vi "HFRR ADV v02.vi"() -> ()   [LabVIEW 2025] (continued)
        n337 = String Length(string=w410) -> (length=w409:i32)
        n338 = Greater?(x=w409, y=1) -> (0:w407:bool)
        n339 = case shown="False" w407 {
          tunnel: w406 -> [w435 _]
          frame False {
            n340 = case shown="False" w435 {
              frame True {
                w436 = "Test Start In Service Mode" ("Tip Strip")
                w437 = T19."Enabled" ("Disabled")
                n341 = property on="Auto Start Test" class="Bool (strict)"("DisabledEnum"=w437, "TipStrip"=w436) -> ()  [unwired: 2 in, 2 out]
                n342 = property on="RUN" class="Bool (strict)"("DisabledEnum"=w437, "TipStrip"=w436) -> ()  [unwired: 2 in, 2 out]
              }
              frame False {
                w438 = "Enter File Name to Start Test" ("Tip Strip")
                w439 = T19."Disabled and Grayed Out" ("Disabled")
                n343 = property on="Auto Start Test" class="Bool (strict)"("DisabledEnum"=w439, "TipStrip"=w438) -> ()  [unwired: 2 in, 2 out]
                n344 = property on="RUN" class="Bool (strict)"("DisabledEnum"=w439, "TipStrip"=w438) -> ()  [unwired: 2 in, 2 out]
              }
            }
          }
          frame True {
            w440 = "" ("Tip Strip")
            w441 = T19."Enabled" ("Disabled")
            n345 = property on="Auto Start Test" class="Bool (strict)"("DisabledEnum"=w441, "TipStrip"=w440) -> ()  [unwired: 2 in, 2 out]
            n346 = property on="RUN" class="Bool (strict)"("DisabledEnum"=w441, "TipStrip"=w440) -> ()  [unwired: 2 in, 2 out]
          }
        }
      }
      event "RUN": Value Change {
        n347 = event-data() -> ()  [unwired: 1 in, 6 out]
        n348 = local read "RUN"() -> (w443:bool)
        n349 = case shown="False" w443 {
          frame False {
            n350 = flat-sequence {
              frame #0 {
                n351 = local write "START TEMP"(FALSE ("START TEMP")) -> ()
              }
              frame #1 {
                n352 = Wait (ms)(milliseconds to wait=u32 1500) -> ()  [unwired: 1 out]
              }
              frame #2 {
                n353 = local write "Humidity 2"(TRUE ("Humidity")) -> ()
              }
              frame #3 {
                n354 = local write "Due Write"("VC;0") -> ()
              }
              frame #4 {
                n355 = Wait (ms)(milliseconds to wait=u32 1500) -> ()  [unwired: 1 out]
              }
              frame #5 {
                w453 = T19."Enabled" ("Disabled")
                (unwired) T25."Imaging" ("Main Dashboard Buttons")
                (unwired) T21."Adv Scar" ("Main Tab")
                w455 = "" ("FILE")
                n356 = local write "measured_stroke"(0.0 ("measured_stroke")) -> ()
                n357 = local write "Due Write"("VC;0") -> ()
                n358 = local write "FILE"(w455) -> ()
                n359 = local write "Batch Ref Num :"(w455) -> ()
                n360 = local write "Fuel Discription :"(w455) -> ()
                n361 = local write "Main Tab"(T4."Adv Scar" ("Main Tab")) -> ()
                n362 = local write "Remarks :"(w455) -> ()
                n363 = local write "Main Dashboard Buttons"(T1."Imaging" ("Main Dashboard Buttons")) -> ()
                n364 = local write "TEST FILE NAM,E SAVED"(FALSE ("TEST FILE NAM,E SAVED")) -> ()
                n365 = property on="Stroke ( mm )" class="WFChart (strict)"("History Data"=cluster{"y":dbl, dbl, "y":dbl}[] []) -> ()  [unwired: 2 in, 2 out]
                n366 = property on="Auto Start Test" class="Bool (strict)"("Visible"=TRUE) -> ()  [unwired: 2 in, 2 out]
                n367 = property on="FRICVALZ 2" class="Bool (strict)"("DisabledEnum"=w453) -> ()  [unwired: 2 in, 2 out]
                n368 = property on="FRICVALZ 4" class="Bool (strict)"("DisabledEnum"=w453) -> ()  [unwired: 2 in, 2 out]
                n369 = property on="FRICVALZ 3" class="Bool (strict)"("DisabledEnum"=w453) -> ()  [unwired: 2 in, 2 out]
              }
            }
          }
          frame True {
            n370 = stacked-sequence {
              frame #0 {
                n371 = local write "FRICVALZ 4"(TRUE ("FRICVALZ 4")) -> ()
                n372 = local write "Due Write"("DAC;200") -> ()
              }
              frame #1 {
              }
              frame #2 {
              }
              frame #3 {
                n373 = Wait (ms)(milliseconds to wait=u32 1000) -> ()  [unwired: 1 out]
              }
              frame #4 {
                n374 = local write "Due Write"("VC;1") -> ()
              }
              frame #5 {
                n375 = Wait (ms)(milliseconds to wait=u32 1000) -> ()  [unwired: 1 out]
              }
              frame #6 {
                n376 = local write "Due Write"("VC;1") -> ()
              }
              frame #7 {
                n377 = Wait (ms)(milliseconds to wait=u32 1500) -> ()  [unwired: 1 out]
              }
              frame #8 {
                w466 = T19."Disabled" ("Disabled")
                n378 = property on="Auto Start Test" class="Bool (strict)"("Visible"=FALSE) -> ()  [unwired: 2 in, 2 out]
                n379 = local write "START TEMP"(TRUE ("START TEMP")) -> ()
                n380 = property on="FRICVALZ 2" class="Bool (strict)"("DisabledEnum"=w466) -> ()  [unwired: 2 in, 2 out]
                n381 = property on="FRICVALZ 4" class="Bool (strict)"("DisabledEnum"=w466) -> ()  [unwired: 2 in, 2 out]
                n382 = property on="FRICVALZ 3" class="Bool (strict)"("DisabledEnum"=w466) -> ()  [unwired: 2 in, 2 out]
              }
            }
          }
        }
      }
      event "run test Calibration": Value Change {
        n383 = event-data() -> ()  [unwired: 1 in, 6 out]
        n384 = local read "run test Calibration"() -> (w468:bool)
        n385 = case shown="False" w468 {
          frame False {
            n386 = flat-sequence {
              frame #0 {
                n387 = local write "START TEMP"(FALSE ("START TEMP")) -> ()
              }
              frame #1 {
                n388 = Wait (ms)(milliseconds to wait=u32 1500) -> ()  [unwired: 1 out]
              }
              frame #2 {
              }
              frame #3 {
                n389 = local write "Due Write"("VC;0") -> ()
              }
              frame #4 {
                n390 = Wait (ms)(milliseconds to wait=u32 1500) -> ()  [unwired: 1 out]
              }
              frame #5 {
                n391 = local write "Due Write"("VC;0") -> ()
                n392 = property on="Tab Control 6" class="TabCtl (strict)"("Visible"=FALSE) -> ()  [unwired: 2 in, 2 out]
                n393 = local write "Friction Force Calibration Result Tab"(enum32{"Calibration Results", "Page 2"}."Calibration Results" ("Friction Force Calibration Result Tab")) -> ()
                n394 = property on="Friction Force Calibration Result Tab" class="TabCtl (strict)"("Visible"=TRUE) -> ()  [unwired: 2 in, 2 out]
              }
            }
          }
          frame True {
            n395 = flat-sequence {
              frame #0 {
                n396 = local write "Due Write"("VC;1") -> ()
              }
              frame #1 {
                n397 = Wait (ms)(milliseconds to wait=u32 1000) -> ()  [unwired: 1 out]
              }
              frame #2 {
                n398 = local write "Due Write"("VC;1") -> ()
              }
              frame #3 {
                n399 = Wait (ms)(milliseconds to wait=u32 2000) -> ()  [unwired: 1 out]
              }
              frame #4 {
                n400 = local write "START TEMP"(TRUE ("START TEMP")) -> ()
                n401 = property on="Tab Control 6" class="TabCtl (strict)"("Visible"=TRUE) -> ()  [unwired: 2 in, 2 out]
                n402 = local write "Friction Force Calibration Result Tab"(enum32{"Calibration Results", "Page 2"}."Calibration Results" ("Friction Force Calibration Result Tab")) -> ()
              }
            }
          }
        }
      }
      event "Auto": Value Change {
        n403 = event-data() -> ()  [unwired: 1 in, 6 out]
        n404 = stacked-sequence {
          frame #0 {
            n405 = local write "FILE"("") -> ()
          }
          frame #1 {
            n406 = Get Date/Time In Seconds() -> (seconds since 1Jan1904=w489:timestamp)
            n407 = Format Into String(format string="%<%m_%d_%Y_%I_%M_%S_%p>T", w489) -> (resulting string=w488:string)  [unwired: 2 in, 1 out]
            n408 = local write "FILE"(w488) -> ()
          }
        }
        n409 = local read "Auto"() -> (w486:bool)
        n410 = Not(x=w486) -> (.not. x?=w485:bool)
        n411 = local write "Auto"(w485) -> ()
      }
      event "Auto Start Temp": Value Change {
        n412 = event-data() -> ()  [unwired: 1 in, 6 out]
        n413 = local read "Auto Start Test"() -> (w492:bool)
        n414 = case shown="False" w492 {
          frame False {
            n415 = stacked-sequence {
              frame #0 {
                n416 = local write "START TEMP"(FALSE ("START TEMP")) -> ()
              }
              frame #1 {
                n417 = Wait (ms)(milliseconds to wait=u32 2000) -> ()  [unwired: 1 out]
              }
              frame #2 {
                n418 = local write "Due Write"("VC;0") -> ()
              }
              frame #3 {
                n419 = Wait (ms)(milliseconds to wait=u32 2000) -> ()  [unwired: 1 out]
              }
              frame #4 {
                w503 = T19."Enabled" ("Disabled")
                (unwired) T25."Imaging" ("Main Dashboard Buttons")
                w504 = "" ("FILE")
                n420 = local write "Main Tab"(T4."Adv Scar" ("Main Tab")) -> ()
                n421 = local write "measured_stroke"(0.0 ("measured_stroke")) -> ()
                n422 = local write "Main Dashboard Buttons"(T1."Imaging" ("Main Dashboard Buttons")) -> ()
                n423 = property on="RUN" class="Bool (strict)"("Visible"=TRUE) -> ()  [unwired: 2 in, 2 out]
                n424 = local write "Due Write"("VC;0") -> ()
                n425 = local write "Humidity 2"(TRUE ("Humidity")) -> ()
                n426 = local write "TEST FILE NAM,E SAVED"(FALSE ("TEST FILE NAM,E SAVED")) -> ()
                n427 = local write "Fuel Discription :"(w504) -> ()
                n428 = local write "Batch Ref Num :"(w504) -> ()
                n429 = local write "Remarks :"(w504) -> ()
                n430 = local write "FILE"(w504) -> ()
                n431 = property on="FRICVALZ 2" class="Bool (strict)"("DisabledEnum"=w503) -> ()  [unwired: 2 in, 2 out]
                n432 = property on="FRICVALZ 4" class="Bool (strict)"("DisabledEnum"=w503) -> ()  [unwired: 2 in, 2 out]
                n433 = property on="FRICVALZ 3" class="Bool (strict)"("DisabledEnum"=w503) -> ()  [unwired: 2 in, 2 out]
              }
            }
          }
          frame True {
            n434 = stacked-sequence {
              frame #0 {
                n435 = local write "Due Write"("DAC;200") -> ()
              }
              frame #1 {
                n436 = Wait (ms)(milliseconds to wait=u32 1000) -> ()  [unwired: 1 out]
              }
              frame #2 {
              }
              frame #3 {
              }
              frame #4 {
                n437 = local write "Due Write"("VC;1") -> ()
              }
              frame #5 {
                n438 = Wait (ms)(milliseconds to wait=u32 1000) -> ()  [unwired: 1 out]
              }
              frame #6 {
                n439 = local write "Due Write"("VC;1") -> ()
              }
              frame #7 {
                n440 = Wait (ms)(milliseconds to wait=u32 1500) -> ()  [unwired: 1 out]
              }
              frame #8 {
                w513 = T19."Disabled" ("Disabled")
                n441 = property on="RUN" class="Bool (strict)"("Visible"=FALSE) -> ()  [unwired: 2 in, 2 out]
                n442 = property on="FRICVALZ 2" class="Bool (strict)"("DisabledEnum"=w513) -> ()  [unwired: 2 in, 2 out]
                n443 = property on="FRICVALZ 4" class="Bool (strict)"("DisabledEnum"=w513) -> ()  [unwired: 2 in, 2 out]
                n444 = property on="FRICVALZ 3" class="Bool (strict)"("DisabledEnum"=w513) -> ()  [unwired: 2 in, 2 out]
                "START TEMP" <- TRUE
              }
            }
          }
        }
      }
      event "FILE", "USERNAME", "USER ID": Mouse Enter {
        n445 = event-data() -> ()  [unwired: 1 in, 4 out]
        n446 = dll-call lib="kernel32.dll" fn="Wow64DisableWow64FsRedirection"("OldValue"=0) -> (error out=w520:errorcluster, "OldValue"=w518:i32)  [unwired: 4 in, 1 out]
        n447 = call <vilib>:"System Exec.vi"("run minimized? (F)"=TRUE, "error in (no error)"=w520, "command line"="C:\\Program Files\\Common Files\\Microsoft Shared\\Ink\\TabTip.exe") -> ("error out"=w519:errorcluster)  [unwired: 5 in, 3 out]
        n448 = dll-call lib="kernel32.dll" fn="Wow64EnableWow64FsRedirection"(error in=w519, "OldValue"=w518) -> ()  [unwired: 4 in, 2 out]
      }
      event "EDIT": Value Change {
        n449 = event-data() -> ()  [unwired: 1 in, 6 out]
        n450 = local read "EDIT"() -> (w521:bool)
        n451 = case shown="False" w521 {
          frame False {
            n452 = control-ref of="This VI"() -> (w538:refnum<vi>)
            n453 = property class="VI"(reference=w538) -> (reference out=w529:refnum<vi>, error out=w533:errorcluster, "Panel"=w537:refnum<vi>)  [unwired: 1 in]
            n454 = property class="Pnl"(reference=w537, error in=w533) -> (reference out=w531:refnum<vi>, error out=w534:errorcluster, "Panes[]"=w536:refnum<vi>[])
            n455 = for {
              tunnel: w536 -> [w544] mode=indexing
              tunnel: T24."Always Off" ("Horizontal Scrollbar Visibility") -> [w543]
              tunnel: w534 -> [w540]
              tunnel: [w539] -> w532
              n456 = property class="Pane"(reference=w544, error in=w540, "HorizScrollbarVisibility"=w543) -> (reference out=w541:refnum<vi>, error out=w542:errorcluster)
              n457 = Close Reference(reference=w541, error in (no error)=w542) -> (error out=w539:errorcluster)
            }
            n458 = Close Reference(reference=w531, error in (no error)=w532) -> (error out=w530:errorcluster)
            n459 = Close Reference(reference=w529, error in (no error)=w530) -> (error out=w524:errorcluster)
            "error out 7" <- w524
            n460 = call <vilib>:"Clear Errors.vi"("error in (no error)"=w524) -> ("error out"=w523:errorcluster)  [unwired: 5 in, 1 out]
            n461 = local write "Service Password enable"(FALSE ("Service Password enable")) -> ()
            n462 = call <userlib>:"Fit VI window to Largest Dec.vi"("error in (no error)"=w523, "border spacing (2 px)"=1) -> ("error out"=w528:errorcluster, "dup VI Ref"=w526:refnum<vi>)  [unwired: 4 in]
            n463 = invoke on="Invoke Node" class="VI" method="FP.Run-Time Position.Maximized"(reference=w526, error in=w528) -> (error out=w527:errorcluster)  [unwired: 2 in, 3 out]
            n464 = call <vilib>:"Clear Errors.vi"("error in (no error)"=w527) -> ()  [unwired: 5 in, 2 out]
          }
          frame True {
          }
        }
      }
      event "Heater Button": Value Change {
        n465 = event-data() -> ()  [unwired: 1 in, 6 out]
        n466 = local read "Heater Button"() -> (w545:bool)
        n467 = case shown="True" w545 {
          frame True {
            n468 = stacked-sequence {
              frame #0 {
                n469 = Wait (ms)(milliseconds to wait=u32 1500) -> ()  [unwired: 1 out]
              }
              frame #1 {
                n470 = local read "Set Temp"() -> (w547:dbl)
                n471 = Number To Fractional String(number=w547, precision (6)=i16 2) -> (F-format string=w550:string)  [unwired: 2 in]
                n472 = Concatenate Strings("ST;" ("Command"), w550) -> (w549:string)
                n473 = local write "Due Write"(w549) -> ()
              }
              frame #2 {
                n474 = Wait (ms)(milliseconds to wait=u32 1500) -> ()  [unwired: 1 out]
              }
              frame #3 {
                n475 = local write "Due Write"("HE;1" ("Command")) -> ()
              }
              frame #4 {
                n476 = Wait (ms)(milliseconds to wait=u32 1500) -> ()  [unwired: 1 out]
              }
              frame #5 {
                n477 = stacked-sequence {
                  frame #0 {
                    n478 = Wait (ms)(milliseconds to wait=u32 1500) -> ()  [unwired: 1 out]
                  }
                  frame #1 {
                    n479 = local read "Set Temp"() -> (w556:dbl)
                    n480 = Number To Fractional String(number=w556, precision (6)=i16 2) -> (F-format string=w559:string)  [unwired: 2 in]
                    n481 = Concatenate Strings("ST;" ("Command"), w559) -> (w558:string)
                    n482 = local write "Due Write"(w558) -> ()
                  }
                  frame #2 {
                    n483 = Wait (ms)(milliseconds to wait=u32 1500) -> ()  [unwired: 1 out]
                  }
                  frame #3 {
                    n484 = local write "Due Write"("HE;1" ("Command")) -> ()
                  }
                  frame #4 {
                    n485 = Wait (ms)(milliseconds to wait=u32 1500) -> ()  [unwired: 1 out]
                  }
                }
              }
            }
          }
          frame False {
            n486 = stacked-sequence {
              frame #0 {
                n487 = Wait (ms)(milliseconds to wait=u32 1500) -> ()  [unwired: 1 out]
              }
              frame #1 {
                n488 = Concatenate Strings("ST;" ("Command"), "0" ("string")) -> (w566:string)
                n489 = local write "Due Write"(w566) -> ()
              }
              frame #2 {
                n490 = Wait (ms)(milliseconds to wait=u32 1500) -> ()  [unwired: 1 out]
              }
              frame #3 {
                n491 = local write "Due Write"("HE;0" ("Command")) -> ()
              }
              frame #4 {
                n492 = Wait (ms)(milliseconds to wait=u32 1500) -> ()  [unwired: 1 out]
              }
            }
          }
        }
      }
      event "Headen Service Button": Value Change {
        n493 = event-data() -> ()  [unwired: 1 in, 6 out]
        n494 = local read "Headen Service Button"() -> (w571:bool)
        n495 = case shown="True" w571 {
          frame False {
            n496 = property on="Password 3" class="Clust (strict)"("Visible"=FALSE) -> ()  [unwired: 2 in, 2 out]
            n497 = property on="Service Password Log" class="Str"("Visible"=FALSE) -> ()  [unwired: 2 in, 2 out]
          }
          frame True {
            n498 = flat-sequence {
              tunnel: [w577] -> w574
              tunnel: w574 -> [w578]
              frame #0 {
                n499 = property on="Password 3" class="Clust (strict)"("Visible"=TRUE) -> ()  [unwired: 2 in, 2 out]
                n500 = property on="Service Password Log" class="Str"("Visible"=TRUE) -> ()  [unwired: 2 in, 2 out]
              }
              frame #1 {
                n501 = call "DIALOG BOX HFRR ADV.vi"() -> ("Continue"=w577:bool)  [unwired: 8 in, 2 out]
              }
              frame #2 {
                n502 = case shown="True" w578 {
                  frame True {
                    n503 = property on="Password 3" class="Clust (strict)"("Visible"=TRUE) -> ()  [unwired: 2 in, 2 out]
                    n504 = property on="Service Password Log" class="Str"("Visible"=TRUE) -> ()  [unwired: 2 in, 2 out]
                  }
                  frame False {
                    n505 = property on="Password 3" class="Clust (strict)"("Visible"=FALSE) -> ()  [unwired: 2 in, 2 out]
                    n506 = property on="Service Password Log" class="Str"("Visible"=FALSE) -> ()  [unwired: 2 in, 2 out]
                  }
                }
              }
            }
          }
        }
      }
      event "Password 3.Service Password": Value Change {
        n507 = event-data() -> ()  [unwired: 1 in, 6 out]
        n508 = Unbundle By Name("Password 3") -> ("Service Password"=w585:string)
        n509 = call <vilib>:"Trim Whitespace.vi"("string"=w585) -> ("trimmed string"=w583:string)  [unwired: 1 in]
        n510 = Equal?(x=w583, y="Service@123") -> (x = y?=w584:bool)
        n511 = case shown="True" w584 {
          selector: w584 -> [w589 w592]
          frame False {
            w588 = FALSE
            n512 = local write "Service Password enable"(w589) -> ()
            n513 = property on="Service Password Log" class="Str"("Visible"=TRUE) -> ()  [unwired: 2 in, 2 out]
            n514 = property on="Service Left" class="Bool (strict)"("Visible"=w588) -> ()  [unwired: 2 in, 2 out]
            n515 = property on="Service Right" class="Bool (strict)"("Visible"=w588) -> ()  [unwired: 2 in, 2 out]
            n516 = property on="Service Bottom" class="Bool (strict)"("Visible"=w588) -> ()  [unwired: 2 in, 2 out]
          }
          frame True {
            w591 = TRUE
            n517 = property on="Service Password Log" class="Str"("Visible"=FALSE) -> ()  [unwired: 2 in, 2 out]
            n518 = property on="Service Left" class="Bool (strict)"("Visible"=w591) -> ()  [unwired: 2 in, 2 out]
            n519 = property on="Service Right" class="Bool (strict)"("Visible"=w591) -> ()  [unwired: 2 in, 2 out]
            n520 = property on="Service Bottom" class="Bool (strict)"("Visible"=w591) -> ()  [unwired: 2 in, 2 out]
            "Service Password enable" <- w592
          }
        }
      }
      event "Sign In": Value Change {
        w594 = FALSE ("Visible")
        n521 = event-data() -> ()  [unwired: 1 in, 6 out]
        n522 = property on="About" class="Clust (strict)"("Visible"=w594) -> ()  [unwired: 2 in, 2 out]
        n523 = property on="Password 3" class="Clust (strict)"("Visible"=w594) -> ()  [unwired: 2 in, 2 out]
        n524 = property on="Service Password Log" class="Str"("Visible"=FALSE) -> ()  [unwired: 2 in, 2 out]
      }
      event "Info": Value Change {
        n525 = event-data() -> ()  [unwired: 1 in, 6 out]
        n526 = local read "Operating System"() -> (w599:string)
        n527 = local read "Firmware Version"() -> (w600:string)
        n528 = local read "Instrument Serial"() -> (w598:string)
        n529 = local read "Workorder"() -> (w602:string)
        n530 = local write "Info"(FALSE) -> ()
        n531 = local read "Runtime"() -> (w601:string)
        n532 = local read "Version"() -> (w603:string)
        n533 = local read "version"() -> (w604:string)
        n534 = Insert Into Array(array=string[] [], new element #1=w604, new element #2=w603, new element #3=w602, new element #4=w601, new element #5=w600, new element #6=w599, new element #7=w598) -> (w597:string[])  [unwired: 1 in]
        n535 = call "ABOUT SCREEN ADV NEW.vi"("Array"=w597) -> ()  [unwired: 10 in, 1 out]
      }
      event "Calibration": Value Change {
        n536 = event-data() -> ()  [unwired: 1 in, 6 out]
        n537 = local read "Calibration"() -> (w607:bool)
        n538 = case shown="False" w607 {
          frame False {
            n539 = property on="Calibration 2" class="TabCtl (strict)"("Visible"=FALSE) -> ()  [unwired: 2 in, 2 out]
            n540 = local write "Cal Password"("" ("Cal Password")) -> ()
          }
          frame True {
            n541 = property on="Calibration 2" class="TabCtl (strict)"("Visible"=TRUE) -> ()  [unwired: 2 in, 2 out]
            n542 = local write "Cal Password"("" ("Cal Password")) -> ()
          }
        }
        n543 = property on="Wrong Password" class="Str"("Visible"=FALSE) -> ()  [unwired: 2 in, 2 out]
      }
      event "Cal Password": Value Change {
        n544 = event-data() -> ()  [unwired: 1 in, 6 out]
        n545 = local read "Cal Password"() -> (w615:string)
        n546 = call <vilib>:"Trim Whitespace.vi"("string"=w615) -> ("trimmed string"=w614:string)  [unwired: 1 in]
        n547 = Equal?(x=w614, y="Cal@321") -> (x = y?=w612:bool)
        n548 = case shown="True" w612 {
          frame False {
            n549 = property on="Wrong Password" class="Str"("Visible"=TRUE) -> ()  [unwired: 2 in, 2 out]
          }
          frame True {
            n550 = property on="Wrong Password" class="Str"("Visible"=FALSE) -> ()  [unwired: 2 in, 2 out]
            n551 = local write "Main Tab"(T4."About" ("Main Tab")) -> ()
            n552 = local write "Cal Password"("" ("Cal Password")) -> ()
            n553 = local write "Main Dashboard Buttons"(T1."About" ("Main Dashboard Buttons")) -> ()
            n554 = property on="Calibration 2" class="TabCtl (strict)"("Visible"=FALSE) -> ()  [unwired: 2 in, 2 out]
            n555 = local write "Calibration"(FALSE ("Calibration")) -> ()
          }
        }
      }
      event "Calibration Selection": Value Change {
        n556 = event-data() -> ()  [unwired: 1 in, 6 out]
        n557 = local read "Calibration Selection"() -> (w624:T10)
        n558 = case shown="\"Stroke Calibration\"" w624 {
          tunnel: [T9."Stroke" ("Main Calibration Tab") T9."Friction" ("Main Calibration Tab") T9."Main" ("Main Calibration Tab") T9."Temperature" ("Main Calibration Tab")] -> w623
          frame "Stroke Calibration" {
          }
          frame "Friction Force Calibration" {
          }
          frame Default {
          }
          frame "Temperature Calibration" {
          }
        }
        n559 = local write "Main Calibration Tab"(w623) -> ()
      }
      event "Back Stroke": Value Change {
        n560 = event-data() -> ()  [unwired: 1 in, 6 out]
        n561 = local write "Main Stroke Tab"(T11."Step 1" ("Main Stroke Tab")) -> ()
        n562 = local write "Main Calibration Tab"(T9."Main" ("Main Calibration Tab")) -> ()
        n563 = local write "Back Stroke"(FALSE ("Back Stroke")) -> ()
        n564 = local write "Calibration Selection"(T10."Default" ("Calibration Selection")) -> ()
      }
      event "Step 2 Back": Value Change {
        n565 = event-data() -> ()  [unwired: 1 in, 6 out]
        n566 = local write "Main Stroke Tab"(T11."Step 1" ("Main Stroke Tab")) -> ()
        n567 = local write "Step 2 Back"(FALSE ("Back Stroke")) -> ()
        n568 = local write "Calibration Selection"(T10."Default" ("Calibration Selection")) -> ()
      }
      event "Step 3 Back": Value Change {
        n569 = event-data() -> ()  [unwired: 1 in, 6 out]
        n570 = local write "Main Stroke Tab"(T11."Step 2" ("Main Stroke Tab")) -> ()
        n571 = local write "Step 3 Back"(FALSE ("Back Stroke")) -> ()
        n572 = local write "Calibration Selection"(T10."Default" ("Calibration Selection")) -> ()
      }
      event "Step 4 Back": Value Change {
        n573 = event-data() -> ()  [unwired: 1 in, 6 out]
        n574 = local write "Main Stroke Tab"(T11."Step 3" ("Main Stroke Tab")) -> ()
        n575 = local write "Step 4 Back"(FALSE ("Back Stroke")) -> ()
        n576 = local write "Calibration Selection"(T10."Default" ("Calibration Selection")) -> ()
      }
      event "Step 5 Back": Value Change {
        n577 = event-data() -> ()  [unwired: 1 in, 6 out]
        n578 = local write "Main Stroke Tab"(T11."Step 4" ("Main Stroke Tab")) -> ()
        n579 = local write "Step 5 Back"(FALSE ("Back Stroke")) -> ()
        n580 = local write "Calibration Selection"(T10."Default" ("Calibration Selection")) -> ()
      }
      event "Step 6 Back": Value Change {
        n581 = event-data() -> ()  [unwired: 1 in, 6 out]
        n582 = local write "Main Stroke Tab"(T11."Step 5" ("Main Stroke Tab")) -> ()
        n583 = local write "Step 6 Back"(FALSE ("Back Stroke")) -> ()
        n584 = local write "Calibration Selection"(T10."Default" ("Calibration Selection")) -> ()
      }
      event "Back Stroke step 7": Value Change {
        n585 = event-data() -> ()  [unwired: 1 in, 6 out]
        n586 = local write "Main Stroke Tab"(T11."Step 5" ("Main Stroke Tab")) -> ()
        n587 = local write "Back Stroke step 7"(FALSE ("Back Stroke")) -> ()
        n588 = local write "Calibration Selection"(T10."Default" ("Calibration Selection")) -> ()
      }
      event "Back Stroke step 8": Value Change {
        n589 = event-data() -> ()  [unwired: 1 in, 6 out]
        n590 = local write "Main Stroke Tab"(T11."Step 7" ("Main Stroke Tab")) -> ()
        n591 = local write "Back Stroke step 8"(FALSE ("Back Stroke")) -> ()
        n592 = local write "Calibration Selection"(T10."Default" ("Calibration Selection")) -> ()
      }
      event "Back Stroke 8": Value Change {
        n593 = event-data() -> ()  [unwired: 1 in, 6 out]
        n594 = local write "MOVE CARRIAGE TO"(1.0 ("MOVE CARRIAGE TO")) -> ()
        n595 = local write "Main Stroke Tab"(T11."Step 1" ("Main Stroke Tab")) -> ()
        n596 = local write "Calibration Selection"(T10."Default" ("Calibration Selection")) -> ()
        n597 = local write "Back Stroke 8"(FALSE ("Back Stroke 8")) -> ()
      }
      event "Continue Stroke": Value Change {
        n598 = event-data() -> ()  [unwired: 1 in, 6 out]
        n599 = local write "Main Stroke Tab"(T11."Step 2" ("Main Stroke Tab")) -> ()
        n600 = local write "Continue Stroke"(FALSE ("Continue Stroke")) -> ()
      }
      event "Continue Stroke step 2": Value Change {
        n601 = event-data() -> ()  [unwired: 1 in, 6 out]
        n602 = local write "Main Stroke Tab"(T11."Step 3" ("Main Stroke Tab")) -> ()
        n603 = local write "Continue Stroke step 2"(FALSE ("Continue Stroke")) -> ()
      }
      event "Continue Stroke step 3": Value Change {
        n604 = event-data() -> ()  [unwired: 1 in, 6 out]
        n605 = local write "Main Stroke Tab"(T11."Step 4" ("Main Stroke Tab")) -> ()
        n606 = local write "Continue Stroke step 3"(FALSE ("Continue Stroke")) -> ()
      }
      event "Continue Stroke step 4": Value Change {
        n607 = event-data() -> ()  [unwired: 1 in, 6 out]
        n608 = local write "Main Stroke Tab"(T11."Step 5" ("Main Stroke Tab")) -> ()
        n609 = local write "Continue Stroke step 4"(FALSE ("Continue Stroke")) -> ()
      }
      event "Continue Stroke step 5": Value Change {
        n610 = event-data() -> ()  [unwired: 1 in, 6 out]
        n611 = local write "Main Stroke Tab"(T11."Step 7" ("Main Stroke Tab")) -> ()
        n612 = local write "Continue Stroke step 5"(FALSE ("Continue Stroke")) -> ()
      }
      event "Continue Stroke step 6": Value Change {
        n613 = event-data() -> ()  [unwired: 1 in, 6 out]
        n614 = local write "Main Stroke Tab"(T11."Step 7" ("Main Stroke Tab")) -> ()
        n615 = local write "Continue Stroke step 6"(FALSE ("Continue Stroke")) -> ()
      }
      event "Continue Stroke step 7": Value Change {
        w672 = FALSE ("0.2mm")
        n616 = event-data() -> ()  [unwired: 1 in, 6 out]
        n617 = local write "0.4 mm"(w672) -> ()
        n618 = local write "0.6 mm"(w672) -> ()
        n619 = local write "1.0 mm"(w672) -> ()
        n620 = local write "1.2 mm"(w672) -> ()
        n621 = local write "0.2 2"(w672) -> ()
        n622 = local write "0.4 2"(w672) -> ()
        n623 = local write "0.6 2"(w672) -> ()
        n624 = local write "0.8 2"(w672) -> ()
        n625 = local write "1.0 2"(w672) -> ()
        n626 = local write "1.2"(w672) -> ()
        n627 = local write "0.2mm"(w672) -> ()
        n628 = local write "0.8mm"(w672) -> ()
        n629 = local write "Main Stroke Tab"(T11."Step 8" ("Main Stroke Tab")) -> ()
        n630 = local write "Continue Stroke step 7"(FALSE ("Continue Stroke")) -> ()
        n631 = local write "Stroke Test Complete"(T12."Test Progress" ("Stroke Test Complete")) -> ()
        "Position Measurment Temp" <- 4.0 ("Position Measurment Temp")
        "Calibration Tare" <- TRUE ("Calibration Tare")
        "MOVE CARRIAGE TO" <- 1.0 ("MOVE CARRIAGE TO")
      }
      event "Continue Stroke step 8": Value Change {
        n632 = event-data() -> ()  [unwired: 1 in, 6 out]
        n633 = local read "LVDT STROKE  Calibration"() -> (w677:dbl)
        n634 = local read "Position Measurment Temp"() -> (w678:dbl)
        n635 = case shown="7" w678 {
          selector: w678 -> [w683 w688 w693 w698 _ w706 w709 w710]
          tunnel: w677 -> [w679 w684 w689 w694 w700 w703 _ _]
          frame 0, Default {
            w681 = TRUE ("0.2mm")
            n636 = Increment(x=w683) -> (x+1=w682:i32)
            n637 = local write "Position Measurment Temp"(w682) -> ()
            n638 = local write "0.2mm"(w681) -> ()
            n639 = local write "0.2 2"(w681) -> ()
            n640 = local write "MOVE CARRIAGE TO"(1.0 ("MOVE CARRIAGE TO")) -> ()
            "Calibration 0.2" <- w679
          }
          frame 1 {
            w686 = TRUE ("0.4 mm")
            n641 = Increment(x=w688) -> (x+1=w687:i32)
            n642 = local write "Calibration 0.4"(w684) -> ()
            n643 = local write "Position Measurment Temp"(w687) -> ()
            n644 = local write "0.4 mm"(w686) -> ()
            n645 = local write "MOVE CARRIAGE TO"(0.6 ("MOVE CARRIAGE TO")) -> ()
            n646 = local write "0.4 2"(w686) -> ()
          }
          frame 2 {
            w691 = TRUE ("0.6 mm")
            n647 = Increment(x=w693) -> (x+1=w692:i32)
            n648 = local write "Calibration 0.6"(w689) -> ()
            n649 = local write "Position Measurment Temp"(w692) -> ()
            n650 = local write "0.6 2"(w691) -> ()
            n651 = local write "0.6 mm"(w691) -> ()
            n652 = local write "MOVE CARRIAGE TO"(0.8 ("MOVE CARRIAGE TO")) -> ()
          }
          frame 3 {
            w695 = TRUE ("0.6 mm")
            n653 = Increment(x=w698) -> (x+1=w697:i32)
            n654 = local write "Position Measurment Temp"(w697) -> ()
            n655 = local write "MOVE CARRIAGE TO"(1.0 ("MOVE CARRIAGE TO")) -> ()
            n656 = local write "0.8mm"(w695) -> ()
            n657 = local write "0.8 2"(w695) -> ()
            "Calibration 0.8" <- w694
          }
          frame 4 {
            w701 = TRUE ("0.6 mm")
            n658 = local write "Position Measurment Temp"(6.0 ("Position Measurment Temp")) -> ()
            n659 = local write "MOVE CARRIAGE TO"(1.0 ("MOVE CARRIAGE TO")) -> ()
            n660 = local write "1.0 mm"(w701) -> ()
            n661 = local write "1.0 2"(w701) -> ()
            "Calibration 1.0" <- w700
          }
          frame 5 {
            w704 = TRUE ("0.6 mm")
            n662 = Increment(x=w706) -> (x+1=w705:i32)
            n663 = local write "Position Measurment Temp"(w705) -> ()
            n664 = local write "1.2 mm"(w704) -> ()
            n665 = local write "1.2"(w704) -> ()
            "Calibration 1.2" <- w703
          }
          frame 6 {
            n666 = Increment(x=w709) -> (x+1=w708:i32)
            n667 = local write "Position Measurment Temp"(w708) -> ()
            n668 = local write "Stroke Test Complete"(T12."Stroke Points Completed" ("Stroke Test Complete")) -> ()
          }
          frame 7 {
            n669 = stacked-sequence {
              tunnel: w710 -> [w711 _ _]
              frame #0 {
                n670 = Increment(x=w711) -> (x+1=w712:i32)
                n671 = local write "Main Stroke Tab"(T11."Step 9" ("Main Stroke Tab")) -> ()
                n672 = local write "Position Measurment Temp"(w712) -> ()
                n673 = Insert Into Array(array=dbl[] [], new element #1=0.2 ("new element/subarray"), new element #2=0.4 ("new element/subarray"), new element #3=0.6 ("new element/subarray"), new element #4=0.8 ("new element/subarray"), new element #5=1.0 ("new element/subarray"), new element #6=1.2 ("new element/subarray")) -> (→"1D stroke":dbl[])  [unwired: 1 in]
                n674 = local read "Calibration 0.2"() -> (w719:dbl)
                n675 = local read "Calibration 0.4"() -> (w718:dbl)
                n676 = local read "Calibration 0.6"() -> (w717:dbl)
                n677 = local read "Calibration 0.8"() -> (w716:dbl)
                n678 = local read "Calibration 1.0"() -> (w715:dbl)
                n679 = local read "Calibration 1.2"() -> (w714:dbl)
                n680 = Insert Into Array(array=dbl[] [], new element #1=w719, new element #2=w718, new element #3=w717, new element #4=w716, new element #5=w715, new element #6=w714) -> (→"Calibrated Voltage Value":dbl[])  [unwired: 1 in]
              }
              frame #1 {
                n681 = local read "calibration values"() -> (w742:dbl[])
                n682 = local read "Calibrated Voltage Value"() -> (w744:dbl[])
                n683 = Index Array(array=w742, index #1=1 ("index"), index #2=3 ("index"), index #3=5 ("index"), index #4=7 ("index"), index #5=9 ("index"), index #6=11 ("index")) -> (element #1=w735:dbl, element #2=w734:dbl, element #3=w733:dbl, element #4=w732:dbl, element #5=w731:dbl, element #6=w730:dbl)
                n684 = local read "1D stroke"() -> (w745:dbl[])
                n685 = for {
                  tunnel: [w754] -> w743 mode=indexing
                  tunnel: w745 -> [w753] mode=indexing
                  tunnel: w744 -> [w752] mode=indexing
                  tunnel: w735 -> [w751]
                  tunnel: w734 -> [w750]
                  tunnel: w733 -> [w749]
                  tunnel: w732 -> [w748]
                  tunnel: w731 -> [w747]
                  tunnel: w730 -> [w746]
                  n686 = formula code="if (stroke == 0.2)\n{\n    if ((voltage >= REF_02 - 0.2) && (voltage <= REF_02 + 0.2))\n        status = 1;\n    else\n        status = 0;\n}\nelse if (stroke == 0.4)\n{\n    if ((voltage >= REF_04 - 0.2) && (voltage <= REF_04 + 0.2))\n        status = 1;\n    else\n        status = 0;\n}\nelse if (stroke == 0.6)\n{\n    if ((voltage >= REF_06 - 0.2) && (voltage <= REF_06 + 0.2))\n        status = 1;\n    else\n        status = 0;\n}\nelse if (stroke == 0.8)\n{\n    if ((voltage >= REF_08 - 0.2) && (voltage <= REF_08 + 0.2))\n        status = 1;\n    else\n        status = 0;\n}\nelse if (stroke == 1.0)\n{\n    if ((voltage >= REF_10 - 1) && (voltage <= REF_10 + 1))\n        status = 1;\n    else\n        status = 0;\n}\nelse if (stroke == 1.2)\n{\n    if ((voltage >= REF_12 - 0.2) && (voltage <= REF_12 + 0.2))\n        status = 1;\n    else\n        status = 0;\n}\nelse\n{\n    status = 0;\n}"("stroke"=w753, "voltage"=w752, "REF_02"=w751, "REF_04"=w750, "REF_06"=w749, "REF_08"=w748, "REF_10"=w747, "REF_12"=w746) -> ("status"=w754:dbl)
                }
                "Status" <- w743
              }
              frame #2 {
                w761 = 1.0
                n687 = local read "Status"() -> (w768:dbl[])
                n688 = Index Array(array=w768) -> (element #1=w767:dbl, element #2=w766:dbl, element #3=w765:dbl, element #4=w764:dbl, element #5=w763:dbl, element #6=w762:dbl)  [unwired: 6 in]
                n689 = Equal?(x=w766, y=w761) -> (x = y?=w759:bool)
                n690 = Equal?(x=w765, y=w761) -> (x = y?=w758:bool)
                n691 = Equal?(x=w764, y=w761) -> (x = y?=w757:bool)
                n692 = Equal?(x=w763, y=w761) -> (x = y?=w756:bool)
                n693 = Equal?(x=w762, y=w761) -> (x = y?=w755:bool)
                n694 = Equal?(x=w767, y=w761) -> (x = y?=w760:bool)
                n695 = case shown="True" w760 {
                  selector: w760 -> [w779 w780]
                  frame True {
                    n696 = local write "Point 1 - 0.2 mm"(w779) -> ()
                    n697 = property on="Point 1 - 0.2 mm" class="Bool"("Caption.Visible"=w779) -> ()  [unwired: 2 in, 2 out]
                  }
                  frame False {
                    n698 = local write "Point 1 - 0.2 mm"(w780) -> ()
                    n699 = property on="Point 1 - 0.2 mm" class="Bool"("Caption.Visible"=w780) -> ()  [unwired: 2 in, 2 out]
                  }
                }
                n700 = case shown="True" w759 {
                  selector: w759 -> [w777 w778]
                  frame True {
                    n701 = local write "Point 2 - 0.4 mm"(w777) -> ()
                    n702 = property on="Point 2 - 0.4 mm" class="Bool"("Caption.Visible"=w777) -> ()  [unwired: 2 in, 2 out]
                  }
                  frame False {
                    n703 = local write "Point 2 - 0.4 mm"(w778) -> ()
                    n704 = property on="Point 2 - 0.4 mm" class="Bool"("Caption.Visible"=w778) -> ()  [unwired: 2 in, 2 out]
                  }
                }
                n705 = case shown="True" w756 {
                  selector: w756 -> [w771 w772]
                  frame True {
                    n706 = local write "Point 5 - 1.0 mm"(w771) -> ()
                    n707 = property on="Point 5 - 1.0 mm" class="Bool"("Caption.Visible"=w771) -> ()  [unwired: 2 in, 2 out]
                  }
                  frame False {
                    n708 = local write "Point 5 - 1.0 mm"(w772) -> ()
                    n709 = property on="Point 5 - 1.0 mm" class="Bool"("Caption.Visible"=w772) -> ()  [unwired: 2 in, 2 out]
                  }
                }
                n710 = case shown="True" w758 {
                  selector: w758 -> [w775 w776]
                  frame True {
                    n711 = local write "Point 3 - 0.6 mm"(w775) -> ()
                    n712 = property on="Point 3 - 0.6 mm" class="Bool"("Caption.Visible"=w775) -> ()  [unwired: 2 in, 2 out]
                  }
                  frame False {
                    n713 = local write "Point 3 - 0.6 mm"(w776) -> ()
                    n714 = property on="Point 3 - 0.6 mm" class="Bool"("Caption.Visible"=w776) -> ()  [unwired: 2 in, 2 out]
                  }
                }
                n715 = case shown="True" w757 {
                  selector: w757 -> [w773 w774]
                  frame True {
                    n716 = local write "Point 4 - 0.8 mm"(w773) -> ()
                    n717 = property on="Point 4 - 0.8 mm" class="Bool"("Caption.Visible"=w773) -> ()  [unwired: 2 in, 2 out]
                  }
                  frame False {
                    n718 = local write "Point 4 - 0.8 mm"(w774) -> ()
                    n719 = property on="Point 4 - 0.8 mm" class="Bool"("Caption.Visible"=w774) -> ()  [unwired: 2 in, 2 out]
                  }
                }
                n720 = case shown="True" w755 {
                  selector: w755 -> [w769 w770]
                  frame True {
                    n721 = local write "Point 6 - 1.2 mm"(w769) -> ()
                    n722 = property on="Point 6 - 1.2 mm" class="Bool"("Caption.Visible"=w769) -> ()  [unwired: 2 in, 2 out]
                  }
                  frame False {
                    n723 = local write "Point 6 - 1.2 mm"(w770) -> ()
                    n724 = property on="Point 6 - 1.2 mm" class="Bool"("Caption.Visible"=w770) -> ()  [unwired: 2 in, 2 out]
                  }
                }
              }
            }
          }
        }
      }
      event "Accept & Save": Value Change {
        n725 = event-data() -> ()  [unwired: 1 in, 6 out]
        n726 = flat-sequence {
          frame #0 {
            n727 = Get Date/Time In Seconds() -> (seconds since 1Jan1904=w783:timestamp)
            n728 = Format Into String(format string="%<%m/%d/%Y %I:%M:%S %p>T", w783) -> (resulting string=w781:string)  [unwired: 2 in, 1 out]
            n729 = local write "STROKE CALIBRATION"(w781) -> ()
          }
          frame #1 {
            n730 = local write "Save Button"(TRUE ("Save Button")) -> ()
          }
          frame #2 {
            n731 = local write "MOVE CARRIAGE TO"(1.0 ("MOVE CARRIAGE TO")) -> ()
            n732 = local write "Main Calibration Tab"(T9."Main" ("Main Calibration Tab")) -> ()
            n733 = local write "Main Stroke Tab"(T11."Step 1" ("Main Stroke Tab")) -> ()
            n734 = local write "Calibration Selection"(T10."Default" ("Calibration Selection")) -> ()
            n735 = local write "Back Stroke 8"(FALSE ("Back Stroke 8")) -> ()
          }
        }
      }
      event "TEMPERATURE STEP Back 1", "TEMPERATURE STEP Back air Temp": Value Change {
        n736 = event-data() -> ()  [unwired: 1 in, 6 out]
        n737 = stacked-sequence {
          frame #0 {
            n738 = local write "Main Calibration Tab"(T9."Main" ("Main Calibration Tab")) -> ()
            n739 = local write "Tab Control 4"(T14."Main" ("Tab Control 4")) -> ()
            n740 = local write "Temperature Selection"(T15."Default" ("Temperature Selection")) -> ()
          }
          frame #1 {
            n741 = Wait (ms)(milliseconds to wait=u32 1000) -> ()  [unwired: 1 out]
            n742 = local write "Calibration Selection"(T10."Default" ("Calibration Selection")) -> ()
          }
          frame #2 {
            n743 = local write "Due Write"("CAL;END" ("Command")) -> ()
          }
          frame #3 {
            n744 = Wait (ms)(milliseconds to wait=u32 2000) -> ()  [unwired: 1 out]
          }
          frame #4 {
            n745 = local write "Due Write"("CAL;END" ("Command")) -> ()
          }
        }
      }
      event "Temperature Continue Step 1": Value Change {
        n746 = event-data() -> ()  [unwired: 1 in, 6 out]
        n747 = stacked-sequence {
          frame #0 {
            n748 = Wait (ms)(milliseconds to wait=u32 1000) -> ()  [unwired: 1 out]
          }
          frame #1 {
            n749 = local write "Due Write"("CAL;START" ("Command")) -> ()
          }
          frame #2 {
            n750 = Wait (ms)(milliseconds to wait=u32 500) -> ()  [unwired: 1 out]
          }
          frame #3 {
            n751 = local write "Due Write"("CAL;START" ("Command")) -> ()
          }
          frame #4 {
            n752 = Wait (ms)(milliseconds to wait=u32 1000) -> ()  [unwired: 1 out]
          }
          frame #5 {
          }
          frame #6 {
          }
          frame #7 {
          }
          frame #8 {
            n753 = local write "Tab Control 4"(T14."Step 2" ("Tab Control 4")) -> ()
          }
        }
      }
      event "Temperature Continue Step air Step 1": Value Change {
        n754 = event-data() -> ()  [unwired: 1 in, 6 out]
        n755 = stacked-sequence {
          frame #0 {
            n756 = Wait (ms)(milliseconds to wait=u32 1000) -> ()  [unwired: 1 out]
          }
          frame #1 {
            n757 = local write "Due Write"("CAL;START" ("Command")) -> ()
          }
          frame #2 {
            n758 = Wait (ms)(milliseconds to wait=u32 1000) -> ()  [unwired: 1 out]
          }
          frame #3 {
            n759 = local write "Due Write"("CAL;START" ("Command")) -> ()
          }
          frame #4 {
          }
          frame #5 {
          }
          frame #6 {
          }
          frame #7 {
          }
          frame #8 {
            n760 = local write "Tab Control 4"(T14."Air Step 2" ("Tab Control 4")) -> ()
          }
        }
      }
      event "Temperature Selection": Value Change {
        n761 = event-data() -> ()  [unwired: 1 in, 6 out]
        n762 = local read "Temperature Selection"() -> (w809:T15)
        n763 = case shown="\"Sample Temperature\"" w809 {
          frame "Air Temperature" {
            n764 = local write "Tab Control 4"(T14."Air Step 1" ("Tab Control 4")) -> ()
          }
          frame "Sample Temperature" {
            n765 = local write "Tab Control 4"(T14."Step 1" ("Tab Control 4")) -> ()
          }
          frame "Default", Default {
          }
        }
      }
      event "Temperature Continue Step 2": Value Change {
        n766 = event-data() -> ()  [unwired: 1 in, 6 out]
        n767 = stacked-sequence {
          frame #0 {
            n768 = stacked-sequence {
              frame #0 {
                n769 = Wait (ms)(milliseconds to wait=u32 1500) -> ()  [unwired: 1 out]
              }
              frame #1 {
                # "CAL;A1;<true_T>"
                n770 = local read "Sensor value"() -> (→"Sample 0deg temp":dbl)
                n771 = local write "Due Write"("CAL;A1;0" ("Command")) -> ()
              }
              frame #2 {
                n772 = Wait (ms)(milliseconds to wait=u32 1500) -> ()  [unwired: 1 out]
              }
              frame #3 {
                # "CAL;A1;<true_T>"
                n773 = local write "Due Write"("CAL;A1;0" ("Command")) -> ()
              }
              frame #4 {
              }
            }
          }
          frame #1 {
            n774 = local write "Tab Control 4"(T14."Step 3" ("Tab Control 4")) -> ()
          }
        }
      }
      event "Temperature Continue Air Step 2": Value Change {
        n775 = event-data() -> ()  [unwired: 1 in, 6 out]
        n776 = stacked-sequence {
          frame #0 {
            n777 = stacked-sequence {
              frame #0 {
                n778 = Wait (ms)(milliseconds to wait=u32 1000) -> ()  [unwired: 1 out]
              }
              frame #1 {
                # "CAL;A1;<true_T>"
                n779 = local write "Due Write"("CAL;A1;0" ("Command")) -> ()
              }
              frame #2 {
                n780 = Wait (ms)(milliseconds to wait=u32 1000) -> ()  [unwired: 1 out]
              }
              frame #3 {
                # "CAL;A1;<true_T>"
                n781 = local write "Due Write"("CAL;A1;0" ("Command")) -> ()
              }
              frame #4 {
                n782 = local read "Sensor value"() -> (→"Air 0deg temp":dbl)
              }
            }
          }
          frame #1 {
            n783 = local write "Tab Control 4"(T14."Air Step 3" ("Tab Control 4")) -> ()
          }
        }
      }
      event "Temperature Continue Step 3": Value Change {
        n784 = event-data() -> ()  [unwired: 1 in, 6 out]
        n785 = stacked-sequence {
          frame #0 {
            n786 = stacked-sequence {
              frame #0 {
                n787 = Wait (ms)(milliseconds to wait=u32 1500) -> ()  [unwired: 1 out]
              }
              frame #1 {
              }
              frame #2 {
              }
              frame #3 {
                # "CAL;A1;<true_T>"
                n788 = local write "Due Write"("CAL;A1;60" ("Command")) -> ()
              }
              frame #4 {
                n789 = Wait (ms)(milliseconds to wait=u32 1000) -> ()  [unwired: 1 out]
              }
              frame #5 {
                # "CAL;A1;<true_T>"
                n790 = local read "Sensor value"() -> (→"Sample 60deg temp":dbl)
                n791 = local write "Due Write"("CAL;A1;60" ("Command")) -> ()
              }
            }
          }
          frame #1 {
            w829 = 0.0
            w830 = 60.0
            n792 = local read "Sample 0deg temp"() -> (w840:dbl)
            n793 = local read "Sample 60deg temp"() -> (w839:dbl)
            n794 = Add(x=w830, y="Temperature diff") -> (x+y=w837:dbl)
            n795 = Subtract(x=w830, y="Temperature diff") -> (x-y=w836:dbl)
            n796 = Add(x=w829, y="Temperature diff") -> (x+y=w835:dbl)
            n797 = Subtract(x=w829, y="Temperature diff") -> (x-y=w834:dbl)
            n798 = In Range and Coerce(upper limit=w837, x=w839, lower limit=w836) -> (In Range?=w833:bool)  [unwired: 1 out]
            n799 = In Range and Coerce(upper limit=w835, x=w840, lower limit=w834) -> (In Range?=w832:bool)  [unwired: 1 out]
            n800 = And(x=w833, y=w832) -> (x .and. y?=w831:bool)
            n801 = case shown="True" w831 {
              frame False {
                n802 = property on="Accept & Save sample Temperature step 4" class="Bool (strict)"("DisabledEnum"=T19."Disabled" ("Disabled")) -> ()  [unwired: 2 in, 2 out]
                n803 = local write "Sample Temperature Calibration"(enum32{"True", "Fail"}."Fail" ("Sample Temperature Calibration  2")) -> ()
              }
              frame True {
                n804 = property on="Accept & Save sample Temperature step 4" class="Bool (strict)"("DisabledEnum"=T19."Enabled" ("Disabled")) -> ()  [unwired: 2 in, 2 out]
                n805 = local write "Sample Temperature Calibration"(enum32{"True", "Fail"}."True" ("Sample Temperature Calibration  2")) -> ()
              }
            }
          }
          frame #2 {
          }
          frame #3 {
          }
          frame #4 {
          }
          frame #5 {
          }
          frame #6 {
            # "CAL;END"
          }
          frame #7 {
          }
          frame #8 {
            # "CAL;END"
          }
          frame #9 {
            n806 = local write "Tab Control 4"(T14."Step 4" ("Tab Control 4")) -> ()
          }
        }
      }
      event "Accept & Save sample Temperature step 4": Value Change {
        n807 = event-data() -> ()  [unwired: 1 in, 6 out]
        n808 = stacked-sequence {
          frame #0 {
            n809 = local write "Due Write"("CAL;SAVE" ("Command")) -> ()
          }
          frame #1 {
            n810 = Wait (ms)(milliseconds to wait=u32 1000) -> ()  [unwired: 1 out]
          }
          frame #2 {
            n811 = local write "Due Write"("CAL;SAVE" ("Command")) -> ()
          }
          frame #3 {
            n812 = Wait (ms)(milliseconds to wait=u32 1000) -> ()  [unwired: 1 out]
          }
          frame #4 {
            n813 = local write "Due Write"("CAL;END" ("Command")) -> ()
          }
          frame #5 {
            n814 = Wait (ms)(milliseconds to wait=u32 1000) -> ()  [unwired: 1 out]
          }
          frame #6 {
            n815 = local write "Due Write"("CAL;END" ("Command")) -> ()
            n816 = local write "Temperature Selection"(T15."Default" ("Temperature Selection")) -> ()
            n817 = local write "Calibration Selection"(T10."Default" ("Calibration Selection")) -> ()
            n818 = local write "Tab Control 4"(T14."Main" ("Tab Control 4")) -> ()
            n819 = local write "Main Calibration Tab"(T9."Temperature" ("Main Calibration Tab")) -> ()
          }
          frame #7 {
            n820 = Get Date/Time In Seconds() -> (seconds since 1Jan1904=w859:timestamp)
            n821 = Format Into String(format string="%<%m/%d/%Y %I:%M:%S %p>T", w859) -> (resulting string=w857:string)  [unwired: 2 in, 1 out]
            n822 = local write "TEMPERATURE CALIBRATION"(w857) -> ()
          }
          frame #8 {
            n823 = local write "Save Button"(TRUE ("Save Button")) -> ()
            n824 = local write "Tab Control 4"(T14."Main" ("Tab Control 4")) -> ()
          }
        }
      }
      event "Accept & Save Air Temperature step 4": Value Change {
        n825 = event-data() -> ()  [unwired: 1 in, 6 out]
        n826 = stacked-sequence {
          frame #0 {
            n827 = local write "Due Write"("CAL;SAVE" ("Command")) -> ()
          }
          frame #1 {
            n828 = Wait (ms)(milliseconds to wait=u32 1000) -> ()  [unwired: 1 out]
          }
          frame #2 {
            n829 = local write "Due Write"("CAL;SAVE" ("Command")) -> ()
          }
          frame #3 {
            n830 = Wait (ms)(milliseconds to wait=u32 1000) -> ()  [unwired: 1 out]
          }
          frame #4 {
            n831 = local write "Due Write"("CAL;END" ("Command")) -> ()
          }
          frame #5 {
            n832 = Wait (ms)(milliseconds to wait=u32 1000) -> ()  [unwired: 1 out]
          }
          frame #6 {
            n833 = local write "Due Write"("CAL;END" ("Command")) -> ()
            n834 = local write "Tab Control 4"(T14."Main" ("Tab Control 4")) -> ()
            n835 = local write "Main Calibration Tab"(T9."Temperature" ("Main Calibration Tab")) -> ()
            n836 = local write "Temperature Selection"(T15."Default" ("Temperature Selection")) -> ()
            n837 = local write "Calibration Selection"(T10."Default" ("Calibration Selection")) -> ()
          }
          frame #7 {
            n838 = Get Date/Time In Seconds() -> (seconds since 1Jan1904=w875:timestamp)
            n839 = Format Into String(format string="%<%m/%d/%Y %I:%M:%S %p>T", w875) -> (resulting string=w874:string)  [unwired: 2 in, 1 out]
            n840 = local write "TEMPERATURE CALIBRATION"(w874) -> ()
          }
          frame #8 {
            n841 = local write "Tab Control 4"(T14."Main" ("Tab Control 4")) -> ()
            n842 = local write "Save Button"(TRUE ("Save Button")) -> ()
          }
        }
      }
      event "Temperature Continue Step 6": Value Change {
        n843 = event-data() -> ()  [unwired: 1 in, 6 out]
        n844 = stacked-sequence {
          frame #0 {
            n845 = stacked-sequence {
              frame #0 {
                n846 = Wait (ms)(milliseconds to wait=u32 1000) -> ()  [unwired: 1 out]
              }
              frame #1 {
              }
              frame #2 {
              }
              frame #3 {
                # "CAL;A1;<true_T>"
                n847 = local write "Due Write"("CAL;A1;60" ("Command")) -> ()
              }
              frame #4 {
                n848 = Wait (ms)(milliseconds to wait=u32 1000) -> ()  [unwired: 1 out]
              }
              frame #5 {
                # "CAL;A1;<true_T>"
                n849 = local write "Due Write"("CAL;A1;60" ("Command")) -> ()
              }
            }
          }
          frame #1 {
            n850 = local read "Sensor value"() -> (→"Air 60deg temp":dbl)
          }
          frame #2 {
          }
          frame #3 {
          }
          frame #4 {
          }
          frame #5 {
          }
          frame #6 {
            # "CAL;END"
          }
          frame #7 {
            w883 = 0.0 ("x")
            w884 = 60.0 ("x")
            n851 = local read "Temperature diff"() -> (w887:dbl)
            n852 = local read "Air 60deg temp"() -> (w886:dbl)
            n853 = local read "Air 0deg temp"() -> (w885:dbl)
            n854 = Add(x=w884, y=w887) -> (x+y=w894:dbl)
            n855 = Subtract(x=w884, y=w887) -> (x-y=w893:dbl)
            n856 = Add(x=w883, y=w887) -> (x+y=w892:dbl)
            n857 = Subtract(x=w883, y=w887) -> (x-y=w891:dbl)
            n858 = In Range and Coerce(upper limit=w894, x=w886, lower limit=w893) -> (In Range?=w890:bool)  [unwired: 1 out]
            n859 = In Range and Coerce(upper limit=w892, x=w885, lower limit=w891) -> (In Range?=w889:bool)  [unwired: 1 out]
            n860 = And(x=w890, y=w889) -> (x .and. y?=w888:bool)
            n861 = case shown="True" w888 {
              frame False {
                n862 = property on="Accept & Save Air Temperature step 4" class="Bool (strict)"("DisabledEnum"=T19."Disabled" ("Disabled")) -> ()  [unwired: 2 in, 2 out]
                n863 = local write "Air Temperature Calibration"(enum32{"True", "Fail"}."Fail" ("Sample Temperature Calibration  2")) -> ()
              }
              frame True {
                n864 = local write "Air Temperature Calibration"(enum32{"True", "Fail"}."True" ("Sample Temperature Calibration  2")) -> ()
                n865 = property on="Accept & Save Air Temperature step 4" class="Bool (strict)"("DisabledEnum"=T19."Enabled" ("Disabled")) -> ()  [unwired: 2 in, 2 out]
              }
            }
          }
          frame #8 {
            # "CAL;END"
          }
          frame #9 {
            n866 = local write "Tab Control 4"(T14."Air Step 4" ("Tab Control 4")) -> ()
          }
        }
      }
      event "Back Stroke step main temperature": Value Change {
        n867 = event-data() -> ()  [unwired: 1 in, 6 out]
        n868 = stacked-sequence {
          frame #0 {
            n869 = Wait (ms)(milliseconds to wait=u32 1000) -> ()  [unwired: 1 out]
          }
          frame #1 {
            # "CAL;END"
            n870 = local write "Due Write"("CAL;END" ("Command")) -> ()
          }
          frame #2 {
            n871 = Wait (ms)(milliseconds to wait=u32 1000) -> ()  [unwired: 1 out]
          }
          frame #3 {
            # "CAL;END"
            n872 = local write "Due Write"("CAL;END" ("Command")) -> ()
          }
          frame #4 {
            n873 = local write "Temperature Selection"(T15."Default" ("Temperature Selection")) -> ()
            n874 = local write "Calibration Selection"(T10."Default" ("Calibration Selection")) -> ()
            n875 = local write "Main Calibration Tab"(T9."Main" ("Main Calibration Tab")) -> ()
            n876 = local write "Tab Control 4"(T14."Main" ("Tab Control 4")) -> ()
          }
        }
      }
      event "TEMPERATURE STEP  Back 4", "TEMPERATURE STEP 1 Back 3", "TEMPERATURE STEP  Back 3", "TEMPERATURE STEP 1 Back 2", "Back Air TEMPERATURE Step 4", "Back SAMPLE TEMPERATURE Step 4": Value Change {
        # "Back Stroke step main temperature"
        n877 = event-data() -> ()  [unwired: 1 in, 6 out]
        n878 = stacked-sequence {
          frame #0 {
            n879 = Wait (ms)(milliseconds to wait=u32 1000) -> ()  [unwired: 1 out]
          }
          frame #1 {
            # "CAL;END"
            n880 = local write "Due Write"("CAL;END" ("Command")) -> ()
          }
          frame #2 {
            n881 = Wait (ms)(milliseconds to wait=u32 1000) -> ()  [unwired: 1 out]
          }
          frame #3 {
            # "CAL;END"
            n882 = local write "Due Write"("CAL;END" ("Command")) -> ()
          }
          frame #4 {
            # "TEMPERATURE STEP  Back 4"
            n883 = local write "Main Calibration Tab"(T9."Temperature" ("Main Calibration Tab")) -> ()
            n884 = local write "Temperature Selection"(T15."Default" ("Temperature Selection")) -> ()
            n885 = local write "Tab Control 4"(T14."Main" ("Tab Control 4")) -> ()
            n886 = local write "Calibration Selection"(T10."Default" ("Calibration Selection")) -> ()
          }
        }
      }
      event "FF BACK", "FF BACK 2", "FF BACK 3", "FF BACK 4", "FF BACK 5", "FF BACK 6": Value Change {
        n887 = event-data() -> ()  [unwired: 1 in, 6 out]
        n888 = stacked-sequence {
          frame #0 {
            n889 = Wait (ms)(milliseconds to wait=u32 1000) -> ()  [unwired: 1 out]
          }
          frame #1 {
            n890 = local write "Due Write"("VC;0") -> ()
          }
          frame #2 {
            n891 = Wait (ms)(milliseconds to wait=u32 1000) -> ()  [unwired: 1 out]
          }
          frame #3 {
            n892 = local write "Due Write"("VC;0") -> ()
          }
          frame #4 {
            w920 = FALSE
            n893 = local write "FF BACK 2"(w920) -> ()
            n894 = local write "FF BACK 3"(w920) -> ()
            n895 = local write "FF BACK 4"(w920) -> ()
            n896 = local write "FF BACK 5"(w920) -> ()
            n897 = local write "FF BACK 6"(w920) -> ()
            n898 = local write "FF BACK"(w920) -> ()
          }
          frame #5 {
